vi "Differentiate - Continuous.vi"(3 "dx/dt 2":dbl=2.5 format="%#_13g", 4 "Input Signal":waveform(dbl)) -> (1 "dx/dt":waveform(dbl))   [LabVIEW 2020]
uses:
  <vilib>/ptbypt/NI_PtbyPt.lvlib
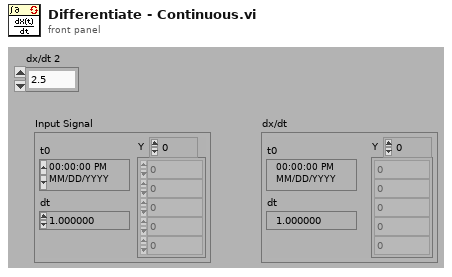
[diagram p1: front panel]
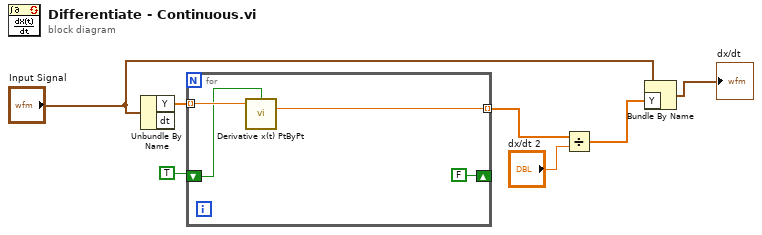
[diagram p0: block diagram]
diagram:
  n1 = Unbundle By Name("Input Signal") -> ("Y"=w5:dbl[])  [unwired: 1 out]
  n2 = for {
    tunnel: w5 -> [w11] mode=indexing
    tunnel: [w8] -> w3 mode=indexing
    shift-right: [FALSE] -> _
    shift-left: TRUE -> [w9]
    n3 = call <vilib>:"Derivative x(t) PtByPt.vi"("initialize"=w9, "x"=w11) -> ("dx/dt"=w8:dbl)  [unwired: 2 in, 1 out]
  }
  n4 = Divide(x=w3, y="dx/dt 2") -> (x/y=w2:dbl[])
  n5 = Bundle By Name(cluster="Input Signal", "Y"=w2) -> (→"dx/dt":waveform(dbl))
